vi "SetMagnification.vi"(8 "error in (no error)":errorcluster, 10 "Sensor.Megnification":i32, 11 "Camera in":refnum<class "Camera.lvclass">) -> (0 "error out":errorcluster, 3 "Camera out":refnum<class "Camera.lvclass">)   [LabVIEW 2020, in "Camera.lvlib" / "Camera.lvclass"]
uses:
  Camera.lvclass
  Camera.lvclass/Camera.ctl
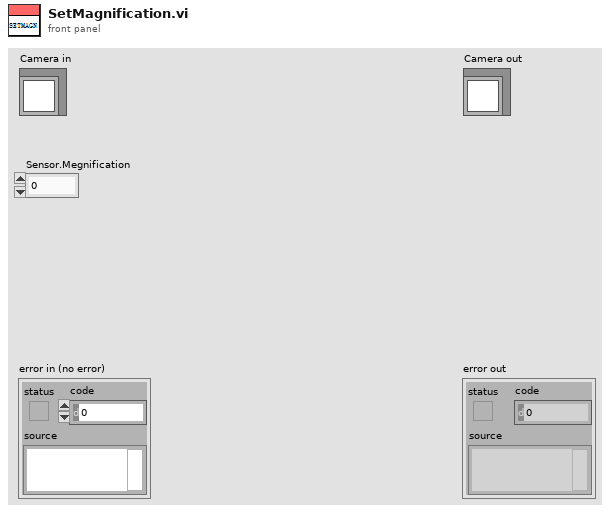
[diagram p1: front panel]
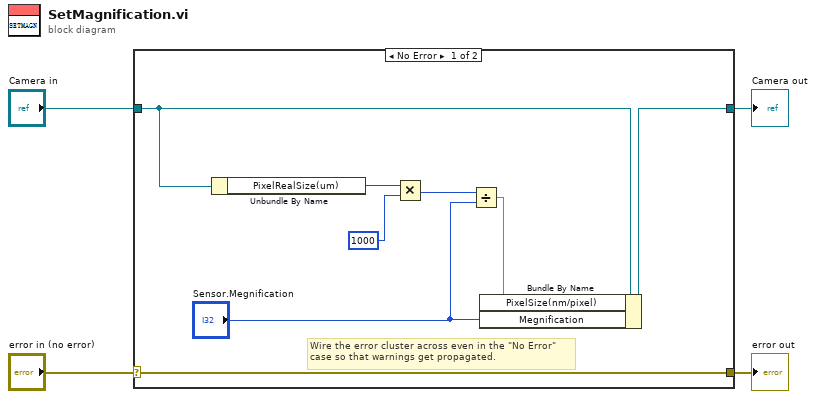
[diagram p0: block diagram]
diagram:
  n1 = case shown="No Error" "error in (no error)" {
    selector: "error in (no error)" -> [w12 w14]
    tunnel: [w12 w14] -> w3
    tunnel: [w11 w13] -> w1
    tunnel: "Camera in" -> [w10 w13]
    frame No Error {
      # "Wire the error cluster across even in the \"No Error\"\ncase so that warnings get propagated."
      n2 = Unbundle By Name(w10) -> ("PixelRealSize(um)"=w9:i32)
      n3 = Multiply(x=w9, y=1000) -> (x*y=w7:i32)
      n4 = Divide(x=w7, y="Sensor.Megnification") -> (x/y=w6:dbl)
      n5 = Bundle By Name(cluster=w10, "PixelSize(nm/pixel)"=w6, "Megnification"="Sensor.Megnification") -> (w11:refnum<class "Camera.lvclass">)
    }
    frame Error {
    }
  }
  "error out" <- w3
  "Camera out" <- w1
